vi "PH_Cont-601k_PSU.Dev Watchdog Device.vi"(0 "VI in":refnum<vi>, 5 "error in (no error)":errorcluster) -> (12 "Charge is allowed":bool, 14 "VI out":refnum<vi>, 15 "Mode":T1, 16 "R2S":bool, 17 "EOC reached?":bool, 18 "Device Error out":errorcluster, 19 "error out":errorcluster)   [LabVIEW 2014, in "PH_Cont-601k_PSU.lvlib"]
uses:
  PH_Cont-601k_PSU.lvlib
  PH_Cont-601k_PSU.Mode.ctl
  PH_Cont-601k_PSU.Device Status.ctl
  instr.lib/pu601k/Continuum PU610K.lvlib
  PH_Basics/PH_Common/PH_Common.lvlib
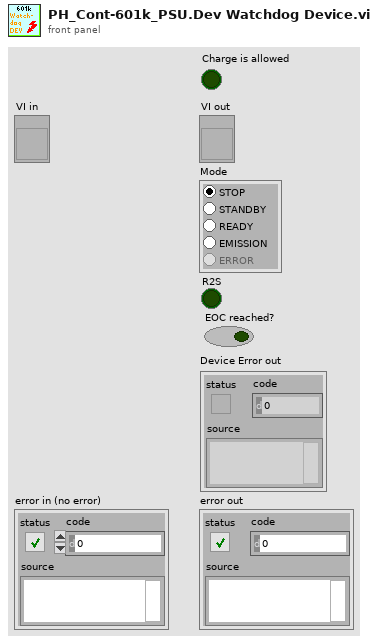
[diagram p1: front panel]
types:
  T1 = typedef "PH_Cont-601k_PSU.lvlib/PH_Cont-601k_PSU.Mode.ctl" = enum32{"STOP", "STANDBY", "READY", "EMISSION", "ERROR"}
  T2 = typedef "PH_Cont-601k_PSU.lvlib/PH_Cont-601k_PSU.Device Status.ctl" = cluster{"State":u16, "Interlocks":cluster{"on/off":bool, "Explanation":string}[], "EOC":u32, "Flashlamp Counter":u32, "error message":string}
  T3 = typedef "PH_Cont-601k_PSU.lvlib/PH_Cont-601k_PSU.i attribute.ctl" = cluster{"GUI Refs":T4, "Interlock":bool, "Service ID applied Voltage":i32, "Device Settings":cluster{"Configuration":T5, "Flash Interval [s]":dbl, "Mode":T1, "Voltage [V]":u16, "Charge":bool, "VISA resource name":refnum<visa-resource-name>}, "Readyness":T6, "Information":cluster{"VISA resource name":refnum<visa-resource-name>, "Tagname Power On":string, "Interlock":cluster{"Instance":string, "Tagname":string}, "Limits [V]":cluster{"Lower":dbl, "Upper":dbl}, "Tagname PSU On":string}, "R2S":bool, "Charge is allowed":bool}
  T4 = typedef "PH_Cont-601k_PSU.lvlib/PH_Cont-601k_PSU.GUI Refs.ctl" = cluster{"Power On":refnum<vi>, "Hard- and Software":refnum<vi>, "Device Status":refnum<vi>, "Device Error":refnum<vi>, "Configuration":refnum<vi>, "Flash Interval [s]":refnum<vi>, "Interlock":refnum<vi>, "Interlock Indicator":refnum<vi>, "Voltage [V]":refnum<vi>, "Readyness":refnum<vi>, "Mode":refnum<vi>, "Reset Error":refnum<vi>, "Expert working":refnum<vi>, "Charge":refnum<vi>, "PSU On":refnum<vi>}
  T5 = typedef "PH_Cont-601k_PSU.lvlib/PH_Cont-601k_PSU.Configuration.ctl" = u16
  T6 = typedef "PH_Cont-601k_PSU.lvlib/PH_Cont-601k_PSU.Readyness.ctl" = cluster{"Program":T7, "Device":T8}
  T7 = typedef "PH_Cont-601k_PSU.lvlib/PH_Cont-601k_PSU.Readyness Program.ctl" = enum32{"OFF", "POWER", "INTERLOCK"}
  T8 = typedef "PH_Cont-601k_PSU.lvlib/PH_Cont-601k_PSU.Readyness Device.ctl" = enum32{"OFF", "CONNECTING", "CONNECTED", "OPERATING", "EOC", "ERROR"}
  T9 = typedef "Continuum PU610K.lvlib/InterlockStatus.ctl" = cluster{"on/off":bool, "Explanation":string}
  T10 = enum16{"Ch intl, Fl intl, QSw intl", "Ch intl, Fl intl, QSw ext", "Ch intl, Fl ext, QSw intl", "Ch intl, Fl ext, QSw ext", "Ch ext, Fl int, QSw int", "Ch ext, Fl int, QSw ext", "Ch ext, Fl ext, QSw int", "Ch ext, Fl ext, QSw ext"}
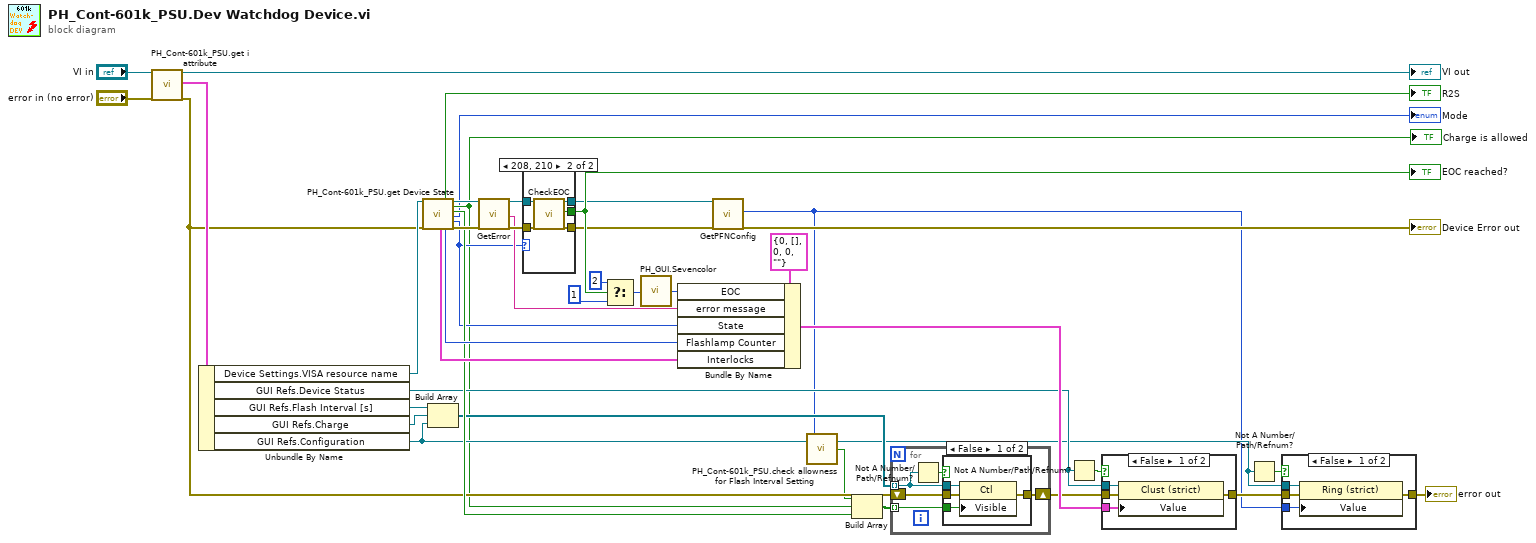
[diagram p0: block diagram]
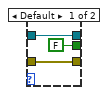
[diagram p2: hidden frame]
diagram:
  n1 = call "PH_Cont-601k_PSU.get i attribute.vi"("i ref in"="VI in", "error in (no error)"="error in (no error)") -> ("i ref out"=→"VI out":refnum<vi>, "i attribute"=w21:T3, "error out"=w11:errorcluster)  [unwired: 15 in]
  n2 = Unbundle By Name(w21) -> ("Device Settings.VISA resource name"=w14:refnum<visa-resource-name>, "GUI Refs.Device Status"=w20:refnum<vi>, "GUI Refs.Flash Interval [s]"=w10:refnum<vi>, "GUI Refs.Charge"=w29:refnum<vi>, "GUI Refs.Configuration"=w15:refnum<vi>)
  n3 = call "PH_Cont-601k_PSU.get Device State.vi"("VISA Refnum in"=w14, "Device Error in"=w11) -> ("Device Status: Interlocks"=w35:T9[], "R2S"=→"R2S":bool, "Device Status: Flashlamp counter"=w34:u32, "VISA Refnum out"=w33:refnum<visa-resource-name>, "Charge is allowed"=w4:bool, "Configuration Change is allowed"=w31:bool, "Mode"=→"Mode":T1, "Device Status: State"=w5:u16, "Device Error out"=w32:errorcluster)  [unwired: 9 in]
  "Charge is allowed" <- w4
  n4 = Build Array(w10, w29, w15) -> (w30:refnum<vi>[])
  n5 = call "GetError.vi"("VISA resource name"=w33, "error in (no error)"=w32) -> ("VISA resource name out"=w25:refnum<visa-resource-name>, "error message"=w24:string, "error out"=w26:errorcluster)  [unwired: 15 in]
  n6 = case shown="208, 210" w5 {
    tunnel: [FALSE ("EOC reached?") w49] -> w40
    tunnel: w26 -> [w43 w48]
    tunnel: w25 -> [w44 w47]
    tunnel: [w44 w46] -> w8
    tunnel: [w43 w45] -> w7
    frame Default {
    }
    frame 208, 210 {
      n7 = call "CheckEOC.vi"("VISA resource name"=w47, "error in"=w48) -> ("VISA resource name out"=w46:refnum<visa-resource-name>, "EOC reached?"=w49:bool, "error out"=w45:errorcluster)  [unwired: 15 in]
    }
  }
  "EOC reached?" <- w40
  n8 = Select(t=2 ("EOC"), s=w40, f=1 ("EOC")) -> (s? t:f=w18:i32)
  n9 = call "PH_GUI.Sevencolor.vi"("State"=w18) -> ("Color Box"=w17:u32)
  n10 = Bundle By Name(cluster=T2 {"State"=0, "Interlocks"=[], "EOC"=0, "Flashlamp Counter"=0, "error message"=""} ("Value"), "EOC"=w17, "error message"=w24, "State"=w5, "Flashlamp Counter"=w34, "Interlocks"=w35) -> (w38:T2)
  n11 = call "GetPFNConfig.vi"("VISA resource name"=w8, "error in"=w7) -> ("PFN Mode"=w3:T10, "error out"=→"Device Error out":errorcluster)  [unwired: 15 in, 1 out]
  n12 = call "PH_Cont-601k_PSU.check allowness for Flash Interval Setting.vi"("Configuration"=w3) -> ("Flash Interval Setting allowed?"=w9:bool)
  n13 = Build Array(w9, w4, w31) -> (w36:bool[])
  n14 = for {
    tunnel: w30 -> [w53] mode=indexing
    shift-right: [w51] -> w37
    shift-left: w11 -> [w52]
    tunnel: w36 -> [w50] mode=indexing
    n15 = Not A Number/Path/Refnum?(number/path/refnum=w53) -> (NaN/Path/Refnum?=w54:bool)
    n16 = case shown="False" w54 {
      tunnel: w52 -> [w58 w59]
      tunnel: [w57 w59] -> w51
      tunnel: w53 -> [w56 _]
      tunnel: w50 -> [w55 _]
      frame False {
        n17 = property class="Ctl"(reference=w56, error in=w58, "Visible"=w55) -> (error out=w57:errorcluster)  [unwired: 1 out]
      }
      frame True {
      }
    }
  }
  n18 = Not A Number/Path/Refnum?(number/path/refnum=w20) -> (NaN/Path/Refnum?=w39:bool)
  n19 = case shown="False" w39 {
    tunnel: w20 -> [w63 _]
    tunnel: w37 -> [w62 w64]
    tunnel: [w61 w64] -> w13
    tunnel: w38 -> [w60 _]
    frame False {
      n20 = property class="Clust (strict)"(reference=w63, error in=w62, "Value"=w60) -> (error out=w61:errorcluster)  [unwired: 1 out]
    }
    frame True {
    }
  }
  n21 = Not A Number/Path/Refnum?(number/path/refnum=w15) -> (NaN/Path/Refnum?=w16:bool)
  n22 = case shown="False" w16 {
    tunnel: w15 -> [w68 _]
    tunnel: w13 -> [w67 w69]
    tunnel: [w66 w69] -> w12
    tunnel: w3 -> [w65 _]
    frame False {
      n23 = property class="Ring (strict)"(reference=w68, error in=w67, "Value"=w65) -> (error out=w66:errorcluster)  [unwired: 1 out]
    }
    frame True {
    }
  }
  "error out" <- w12
